vi "Factorial square sum.vi"() -> ()   [LabVIEW 2016]
uses:
  <vilib>/gmath/NI_Gmath.lvlib
panel:
  out "ans":dbl
  in  "x":dbl
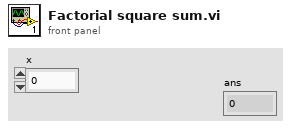
[diagram p1: front panel]
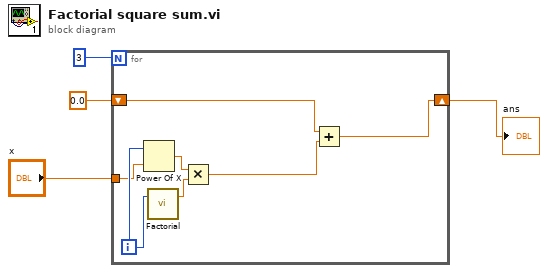
[diagram p0: block diagram]
diagram:
  n1 = for {
    N: 3 -> [_]
    tunnel: "x" -> [w8]
    shift-right: [w5] -> w1
    shift-left: 0.0 -> [w6]
    i -> [w9]
    n2 = Power Of X(1:w8, 2:w9) -> (0:w10:dbl)
    n3 = call <vilib>:"Factorial.vi"("n"=w9) -> ("n!"=w11:dbl)  [unwired: 2 in]
    n4 = Multiply(x=w10, y=w11) -> (x*y=w7:dbl)
    n5 = Add(x=w6, y=w7) -> (x+y=w5:dbl)
  }
  "ans" <- w1
